vi "DAQNavi Write (Digtial 1D U8 NChan 1Samp).vi"(8 "error in (no error)":errorcluster, 9 "timeout":dbl=10.0, 10 "data":u8[](array[numeric]), 11 "task in":i32) -> (0 "error out":errorcluster, 2 "number of samples written per channel":u32, 3 "task out":i32)   [LabVIEW 2020]
uses:
  DAQNavi_LV.dll
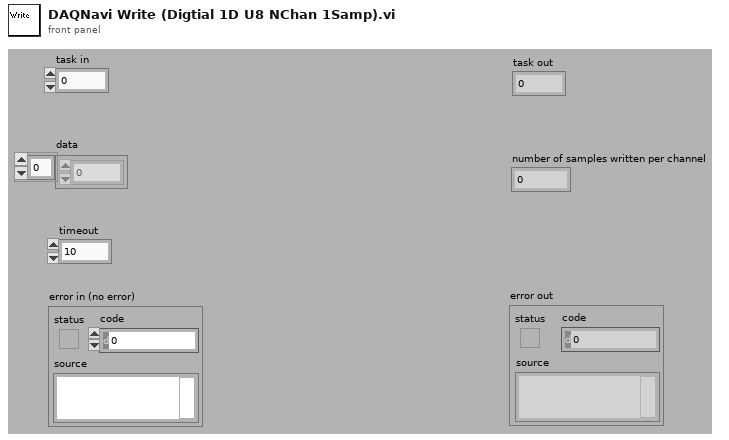
[diagram p1: front panel]
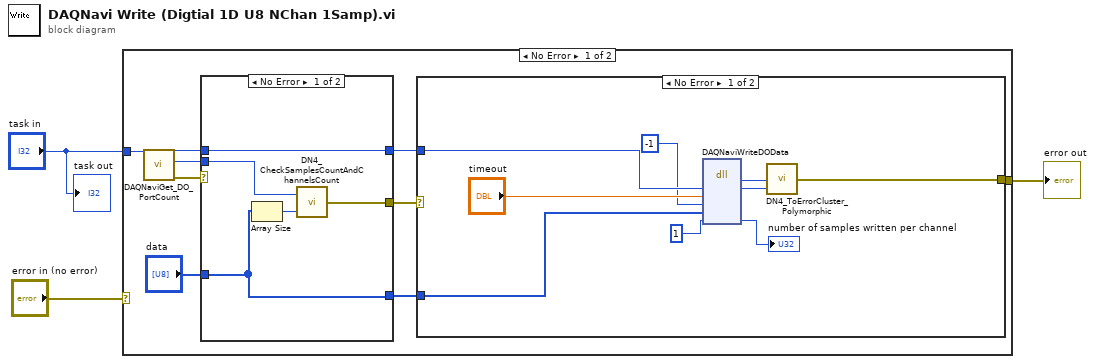
[diagram p0: block diagram]
diagram:
  n1 = case shown="No Error" "error in (no error)" {
    selector: "error in (no error)" -> [_ w31]
    tunnel: [w6 w31] -> w2
    tunnel: "task in" -> [w9 _]
    frame No Error {
      n2 = call "DAQNaviGet_DO_PortCount.vi"("task in"=w9) -> ("error out"=w12:errorcluster, "port count"=w11:i32, "task out"=w10:i32)  [unwired: 1 in, 7 out]
      n3 = case shown="No Error" w12 {
        selector: w12 -> [_ w20]
        tunnel: w11 -> [w16 _]
        tunnel: [w13 w20] -> w8
        tunnel: [w17 w19] -> w7
        tunnel: w10 -> [w17 w19]
        tunnel: "data" -> [w14 w18]
        tunnel: [w14 w18] -> w4
        frame No Error {
          n4 = Array Size(array=w14) -> (size(s)=w15:i32)
          n5 = call "DN4_CheckSamplesCountAndChannelsCount.vi"("samples count"=w15, "channel count"=w16) -> ("error out"=w13:errorcluster)
        }
        frame Error {
        }
      }
      n6 = case shown="No Error" w8 {
        selector: w8 -> [_ w30]
        tunnel: w7 -> [w29 _]
        tunnel: [w28 w30] -> w6
        tunnel: w4 -> [w23 _]
        frame No Error {
          n7 = dll-call lib="DAQNavi_LV.dll" fn="DAQNaviWriteDOData"("taskID"=w29, "timeout"="timeout", "portBit"=-1, "portData"=w23, "samples"=u32 1) -> ("return type"=w25:i32, "taskID"=w22:i32, "samples"=→"number of samples written per channel":u32)  [unwired: 6 in, 2 out]
          n8 = call "DN4_ToErrorCluster_Polymorphic.vi"("task id"=w22, "error code"=w25) -> ("error out"=w28:errorcluster)  [unwired: 3 out]
        }
        frame Error {
        }
      }
    }
    frame Error {
    }
  }
  "error out" <- w2
  "task out" <- "task in"
